vi "List Class Paths.vi"(8 "error in (no error)":errorcluster) -> (0 "error out":errorcluster, 2 "Class Paths":path[](array[path]), 3 "Class Names":string[](array[string]))   [LabVIEW 2020, in "ClassLoader.lvlib"]
doc: "List all cached class names and paths.\n\nThis VI does not automatically load data. Front-load before calling this VI!"
uses:
  ClassLoader.lvlib
  Sub/Cache/Cache_Path Global.vi
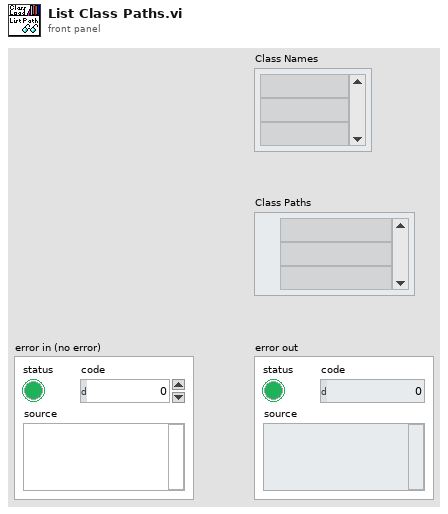
[diagram p1: front panel]
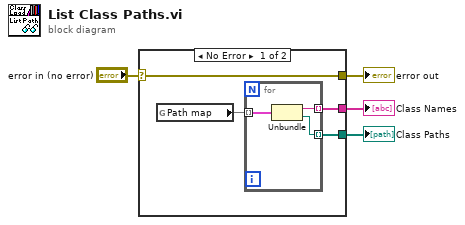
[diagram p0: block diagram]
diagram:
  n1 = case shown="No Error" "error in (no error)" {
    selector: "error in (no error)" -> [w5 w12]
    tunnel: [w7 _] -> w4
    tunnel: [w6 _] -> w3
    tunnel: [w5 w12] -> w1
    frame No Error {
      n2 = global read "Cache_Path Global.vi" "Path map"() -> (w8:map{string, path})
      n3 = for {
        tunnel: w8 -> [w11] mode=indexing
        tunnel: [w10] -> w7 mode=indexing
        tunnel: [w9] -> w6 mode=indexing
        n4 = Unbundle(w11) -> ("key"=w10:string, "value"=w9:path)
      }
    }
    frame Error {
    }
  }
  "error out" <- w1
  "Class Paths" <- w3
  "Class Names" <- w4
